vi "test - Time Comparison - 1.vi"(8 "error in (no error)":errorcluster, 11 "TestCase in":refnum<class "Time Filter Tester.lvclass">) -> (0 "error out":errorcluster, 3 "TestCase out":refnum<class "Time Filter Tester.lvclass">)   [LabVIEW 2016, in "Time Filter Tester.lvclass"]
uses:
  Time Filter Tester.lvclass
  Time Filter Tester.lvclass/Time Filter Tester.ctl
  <vilib>/addons/_JKI Toolkits/VI Tester/TestCase.llb/TestCase.lvclass
  Core/Assert API Components/Filter Configurations/Time Filters/Time Filters.lvclass
  C:/Program Files (x86)/National Instruments/LabVIEW 2016/vi.lib/addons/_JKI Toolkits/VI Tester/TestCase.llb/TestCase.lvclass
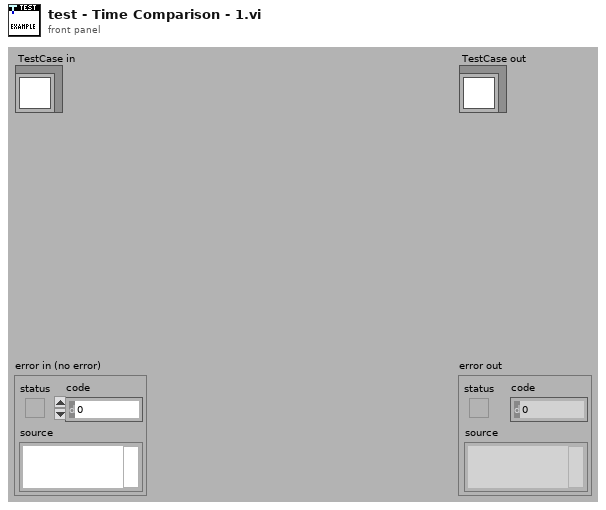
[diagram p1: front panel]
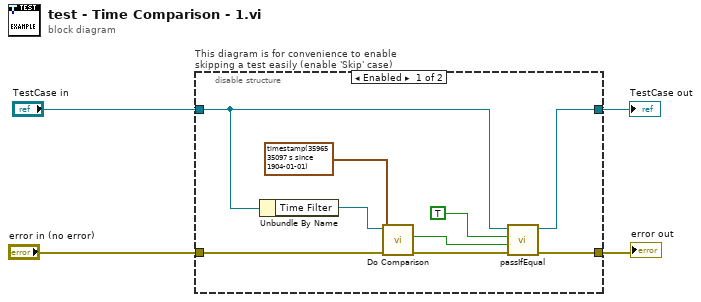
[diagram p0: block diagram]
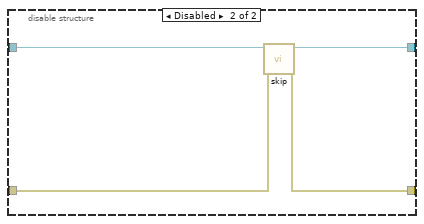
[diagram p2: hidden frame]
diagram:
  n1 = disable-structure "This diagram is for convenience to enable skipping a test easily (enable 'Skip' case)" shown="Enabled" {
    disable-tunnel: "TestCase in" -> [w11 w17]
    disable-tunnel: [w13 w15] -> w1
    disable-tunnel: [w12 w16] -> w3
    disable-tunnel: "error in (no error)" -> [w8 w14]
    frame Enabled {
      n2 = Unbundle By Name(w11) -> ("Time Filter"=w10:refnum<class "Time Filters.lvclass">)
      n3 = call "Do Comparison.vi"("error in (no error)"=w8, "Compare Timestamp"=timestamp(3596535097.131794 s since 1904-01-01), "Time Filters in"=w10) -> ("error out"=w7:errorcluster, "Filtered"=w6:bool)  [unwired: 7 in]
      n4 = call-dynamic "passIfEqual.vi"("error in (no error)"=w7, "y"=w6, "x"=TRUE, "TestCase in"=w11) -> ("error out"=w12:errorcluster, "TestCase out"=w13:refnum<class "Time Filter Tester.lvclass">)  [unwired: 6 in]
    }
    frame Disabled {
      # "skip test result while test is under development"
      n5 = call <vilib>:"skip.vi"("error in (no error)"=w14, "TestCase in"=w17) -> ("error out"=w16:errorcluster, "TestCase out"=w15:refnum<class "Time Filter Tester.lvclass">)  [unwired: 8 in]
    }
  }
  "error out" <- w3
  "TestCase out" <- w1
